vi "Get Stylesheet MIME Type from File Extension.vi"(8 "error in":errorcluster, 10 "Stylesheet URL":string) -> (0 "error out":errorcluster, 2 "MIME type":string)   [LabVIEW 2013]
uses:
  <userlib>/_OpenG.lib/file/file.llb/Strip Path Extension - String__ogtk.vi
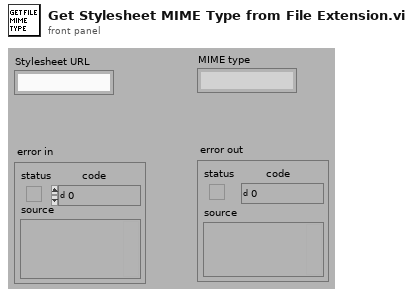
[diagram p1: front panel]
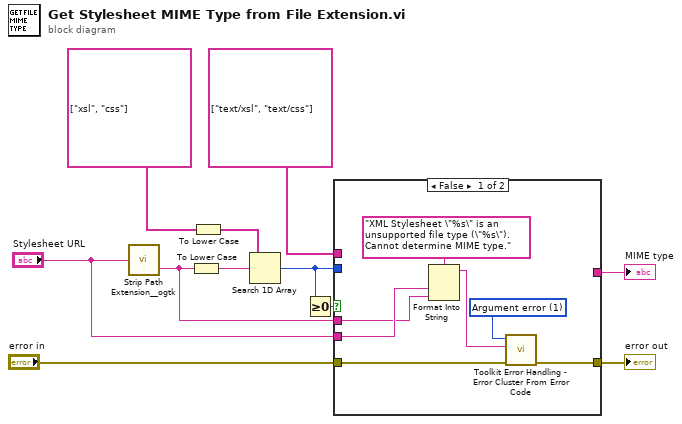
[diagram p0: block diagram]
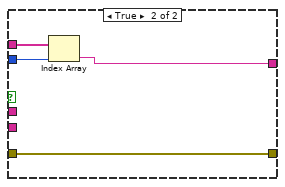
[diagram p2: hidden frame]
diagram:
  n1 = call-poly <userlib>:"Strip Path Extension__ogtk.vi"("path"="Stylesheet URL") -> ("extension"=w1:string)  [unwired: 1 out]
  n2 = To Lower Case(string=w1) -> (all lower case string=w9:string)
  n3 = To Lower Case(string=string[] ["xsl", "css"]) -> (all lower case string=w10:string[])
  n4 = Search 1D Array(1D array=w10, element=w9) -> (index of element=w7:i32)  [unwired: 1 in]
  n5 = Greater Or Equal To 0?(x=w7) -> (x >= 0?=w3:bool)
  n6 = case shown="False" w3 {
    tunnel: string[] ["text/xsl", "text/css"] -> [_ w22]
    tunnel: w7 -> [_ w21]
    tunnel: [w17 w20] -> w6
    tunnel: "error in" -> [w18 w20]
    tunnel: [_ w19] -> w4
    tunnel: "Stylesheet URL" -> [w16 _]
    tunnel: w1 -> [w15 _]
    frame False {
      w12 = 1 items=["No error", "Argument error", "Memory is full", "Out of zone", "End of file", "File already open", "Generic file I/O error", "File not found", "File permission error", "Disk is full", "Duplicate path", "Too many files open", "System feature not enabled", "Resource file not found", "Cannot add resource", "Resource not found", "Image not found", "Image memory error", "Pen does not exist", "Config type invalid", "Config token not found", "Config parse error", "Config memory error", "Bad external code format", "Bad external code offset", "External code not present", "Null window", "Destroy window error", "Null menu", "Print aborted", "Bad print record", "Print driver error", "Windows error during printing", "Memory error during printing", "Print dialog error", "Generic print error", "Invalid device refnum", "Device not found", "Device parameter error", "Device unit error", "Cannot open device", "Device call aborted", "Generic error", "Cancelled by user", "Object ID too low", "Object ID too high", "Object not in heap", "Unknown heap", "Unknown object (invalid DefProc)", "Unknown object (DefProc not in table)", "Message out of range", "Invalid (null) method", "Unknown message", "Manager call not supported", "Bad address", "Network operation in progress", "Network operation timed out", "Connection is busy", "Network attribute not supported", "Network error", "Address in use", "System out of memory", "Connection aborted", "Connection refused", "Not connected", "Already connected", "Connection closed", "Initialization error (interapplication manager)", "Bad occurrence", "Wait on unbound occurrence handler", "Occurrence queue overflow", "Datalog type conflict", "Unused", "Unrecognized type (interapplication manager)", "Memory corrupt", "Failed to make temporary DLL", "Old CIN version", "Drag socket not found", "Failed to load drop-object", "Failed to register OLE object", "Failed to release OLE object", "Format specifier type mismatch", "Unknown format specifier", "Too few format specifiers", "Too many format specifiers", "Scan failed", "Newer CIN version", "Error converting to variant", "Runtime menu error", "Password tampered", "Variant attribute not found", "Incompatible variant data type", "Event data is not available", "Event Store is not present", "Occurrence is not found", "Event Queue is not created", "Event info is not available", "Refnum passed is NULL", "Error retrieving Class GUID", "Error retrieving CoClass GUID", "Error retrieving TypeLib GUID.", "Bad built application magic bytes.", "Specific driver is different from the specific driver associated with the Logical Name.", "There is no session opened to the class driver.", "Max Error", "MAX - Error with config objects", "MAX - Error loading configuration", "MAX - Group not supported"]
      n7 = Format Into String(format string="XML Stylesheet \"%s\" is an unsupported file type (\"%s\").  Cannot determine MIME type.", w16, w15) -> (resulting string=w13:string)  [unwired: 2 in, 1 out]
      n8 = call "Toolkit Error Handling - Error Cluster From Error Code.vi"("error in"=w18, "error message (\"\")"=w13, "error code (0)"=w12) -> ("error out"=w17:errorcluster)  [unwired: 6 in]
    }
    frame True {
      n9 = Index Array(array=w22, index=w21) -> (element=w19:string)
    }
  }
  "error out" <- w6
  "MIME type" <- w4
